vi "getpath.vi"() -> (3 "stripped path":path)   [LabVIEW 2013]
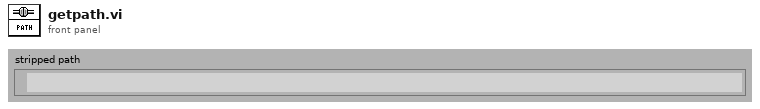
[diagram p1: front panel]
types:
  T1 = enum32{"invalid app kind", "Development System", "Run Time System", "Student Edition", "Embedded LabVIEW", "Evaluation", "Custom"}
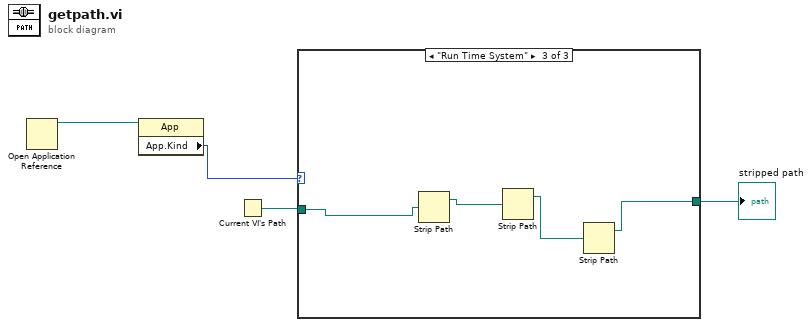
[diagram p0: block diagram]
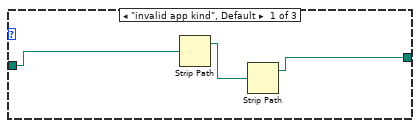
[diagram p2: hidden frame]
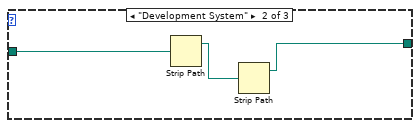
[diagram p3: hidden frame]
diagram:
  n1 = Open Application Reference() -> (3:w4:refnum<vi>)  [unwired: 4 in, 1 out]
  n2 = property class="App"(reference=w4) -> ("App.Kind"=w3:T1)  [unwired: 1 in, 2 out]
  n3 = Current VI's Path() -> (path=w2:path)
  n4 = case shown="\"Run Time System\"" w3 {
    tunnel: w2 -> [w6 w10 w14]
    tunnel: [w5 w8 w11] -> w1
    frame "invalid app kind", Default {
      n5 = Strip Path(path=w6) -> (stripped path=w7:path)  [unwired: 1 out]
      n6 = Strip Path(path=w7) -> (stripped path=w5:path)  [unwired: 1 out]
    }
    frame "Development System" {
      n7 = Strip Path(path=w10) -> (stripped path=w9:path)  [unwired: 1 out]
      n8 = Strip Path(path=w9) -> (stripped path=w8:path)  [unwired: 1 out]
    }
    frame "Run Time System" {
      n9 = Strip Path(path=w14) -> (stripped path=w13:path)  [unwired: 1 out]
      n10 = Strip Path(path=w13) -> (stripped path=w12:path)  [unwired: 1 out]
      n11 = Strip Path(path=w12) -> (stripped path=w11:path)  [unwired: 1 out]
    }
  }
  "stripped path" <- w1
